vi "ProdaNG.Tree.ProcessSteps.Add.vi"(6 "WabcoPartId":i32, 7 "Tree":refnum<vi>, 8 "error in (no error)":errorcluster, 9 "ProcId":i32, 10 "ProcSteps in":T1[](array[typedef])) -> (0 "error out":errorcluster, 2 "ProcSteps out":T1[](array[typedef]))   [LabVIEW 2016]
uses:
  Controls/ProdaNG.ProcessStep.ctl
  ProdaNG.Configurator.Glb.vi
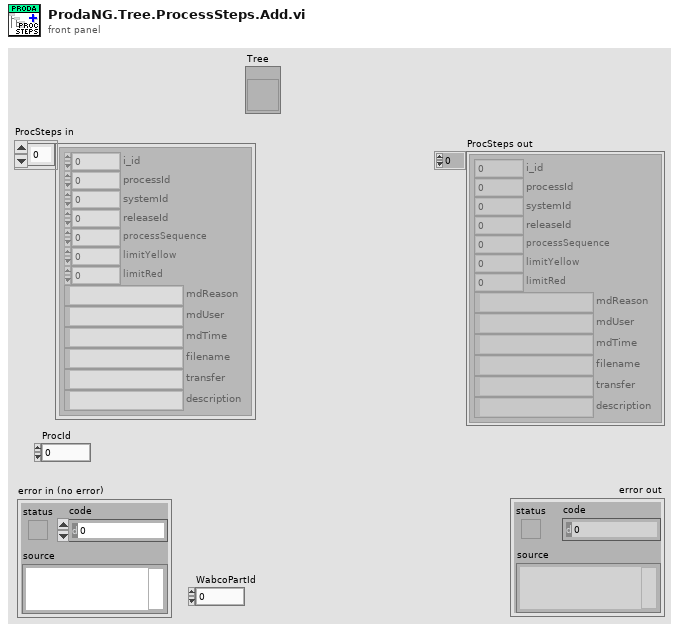
[diagram p1: front panel]
types:
  T1 = typedef "ProdaNG.ProcessStep.ctl" = cluster{"i_id":i32, "processId":i32, "systemId":i32, "releaseId":i32, "processSequence":i32, "limitYellow":dbl, "limitRed":dbl, "mdReason":string, "mdUser":string, "mdTime":string, "filename":string, "transfer":string, "description":string}
  T2 = typedef "ProdaNG.System.ctl" = cluster{"i_id":i32, "description":string}
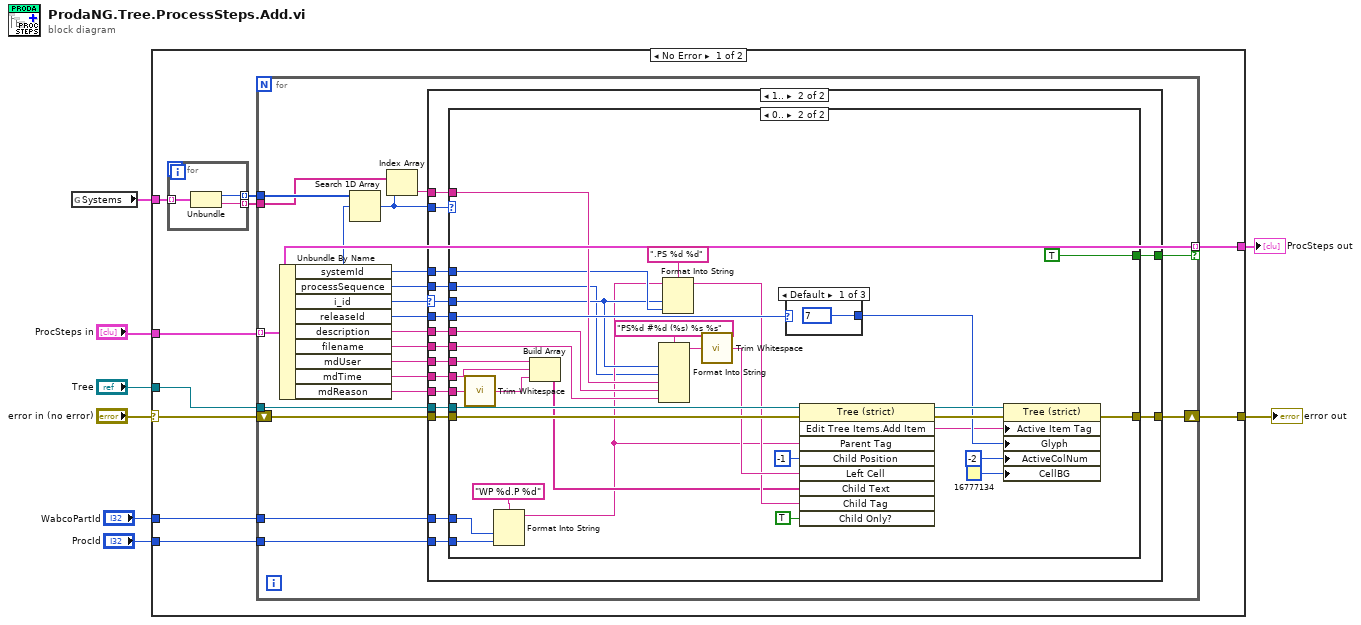
[diagram p0: block diagram]
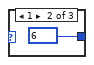
[diagram p4: hidden frame]
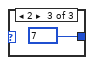
[diagram p5: hidden frame]
diagram:
  n1 = global read "ProdaNG.Configurator.Glb.vi" "Systems"() -> (w2:T2[])
  n2 = case shown="No Error" "error in (no error)" {
    selector: "error in (no error)" -> [w18 w97]
    tunnel: [w16 w97] -> w7
    tunnel: "Tree" -> [w17 _]
    tunnel: "ProcSteps in" -> [w15 _]
    tunnel: [w14 _] -> w5
    tunnel: w2 -> [w13 _]
    tunnel: "ProcId" -> [w10 _]
    tunnel: "WabcoPartId" -> [w9 _]
    frame No Error {
      n3 = for {
        tunnel: w13 -> [w96] mode=indexing
        tunnel: [w95] -> w12 mode=indexing
        tunnel: [w94] -> w11 mode=indexing
        n4 = Unbundle(w96) -> ("i_id"=w95:i32, "description"=w94:string)
      }
      n5 = for {
        tunnel: w17 -> [w37]
        tunnel: w15 -> [w29] mode=indexing
        shift-right: [w31] -> w16
        shift-left: w18 -> [w38]
        tunnel: [w29] -> w14 mode=indexing if=w28
        tunnel: w12 -> [w27]
        tunnel: w11 -> [w26]
        tunnel: w10 -> [w22]
        tunnel: w9 -> [w21]
        n6 = Unbundle By Name(w29) -> ("systemId"=w25:i32, "processSequence"=w19:i32, "i_id"=w30:i32, "releaseId"=w35:i32, "description"=w36:string, "filename"=w23:string, "mdUser"=w34:string, "mdTime"=w33:string, "mdReason"=w32:string)
        n7 = Search 1D Array(1D array=w27, element=w25) -> (index of element=w24:i32)  [unwired: 1 in]
        n8 = Index Array(array=w26, index=w24) -> (element=w20:string)
        n9 = case shown="1.." w30 {
          selector: w30 -> [_ w51]
          tunnel: w38 -> [w39 w56]
          tunnel: w37 -> [_ w55]
          tunnel: w36 -> [_ w49]
          tunnel: w35 -> [_ w54]
          tunnel: w34 -> [_ w53]
          tunnel: w33 -> [_ w45]
          tunnel: w32 -> [_ w52]
          tunnel: [w39 w46] -> w31
          tunnel: [_ w50] -> w28
          tunnel: w20 -> [_ w48]
          tunnel: w25 -> [_ w47]
          tunnel: w24 -> [_ w44]
          tunnel: w23 -> [_ w43]
          tunnel: w22 -> [_ w42]
          tunnel: w21 -> [_ w41]
          tunnel: w19 -> [_ w40]
          frame 0, Default {
          }
          frame 1.. {
            n10 = case shown="0.." w44 {
              tunnel: w56 -> [w57 w90]
              tunnel: w55 -> [_ w89]
              tunnel: w54 -> [_ w87]
              tunnel: w53 -> [_ w66]
              tunnel: w52 -> [_ w64]
              tunnel: w51 -> [_ w73]
              tunnel: [_ TRUE] -> w50
              tunnel: w49 -> [_ w85]
              tunnel: w48 -> [_ w84]
              tunnel: w47 -> [_ w75]
              tunnel: [w57 w78] -> w46
              tunnel: w45 -> [_ w62]
              tunnel: w43 -> [_ w74]
              tunnel: w42 -> [_ w70]
              tunnel: w41 -> [_ w61]
              tunnel: w40 -> [_ w59]
              frame Default {
              }
              frame 0.. {
                n11 = call <vilib>:"Trim Whitespace.vi"("string"=w64) -> ("trimmed string"=w65:string)  [unwired: 1 in]
                n12 = Format Into String(format string="WP %d.P %d", w61, w70) -> (resulting string=w60:string)  [unwired: 2 in, 1 out]
                n13 = Build Array(w66, w62, w65) -> (w63:string[])
                n14 = Format Into String(format string="PS%d #%d (%s) %s %s", w73, w59, w84, w85, w74) -> (resulting string=w83:string)  [unwired: 2 in, 1 out]
                n15 = Format Into String(format string=".PS %d %d", initial string=w60, w73, w75) -> (resulting string=w68:string)  [unwired: 1 in, 1 out]
                n16 = call <vilib>:"Trim Whitespace.vi"("string"=w83) -> ("trimmed string"=w69:string)  [unwired: 1 in]
                n17 = case shown="Default" w87 {
                  tunnel: [7 6 7] -> w77
                  frame Default {
                  }
                  frame 1 {
                  }
                  frame 2 {
                  }
                }
                n18 = invoke class="Tree (strict)" method="Edit Tree Items.Add Item"(reference=w89, error in=w90, "Parent Tag"=w60, "Child Position"=-1, "Left Cell"=w69, "Child Text"=w63, "Child Tag"=w68, "Child Only?"=TRUE) -> (reference out=w80:refnum<vi>, error out=w79:errorcluster, "Edit Tree Items:Add Item"=w76:string)  [unwired: 1 in, 6 out]
                n19 = property class="Tree (strict)"(reference=w80, error in=w79, "Active Item Tag"=w76, "Glyph"=w77, "ActiveColNum"=-2 ("Active Cell:Active Column Number"), "CellBG"=u32 16777134) -> (error out=w78:errorcluster)  [unwired: 1 out]
              }
            }
          }
        }
      }
    }
    frame Error {
    }
  }
  "error out" <- w7
  "ProcSteps out" <- w5
